vi "Get Attributes.vi"(7 "Tree ID":string, 8 "Error In":errorcluster, 10 "Attributes Names":string[](array[string]), 11 "Tree Manager":T1) -> (0 "Error Out":errorcluster, 1 "Attribute Value":variant[](array[variant]), 2 "Found?":bool[](array[boolean]), 3 "Tree Manager":T1)   [LabVIEW 2020, in "NI_VIAnCFGDataStructure.lvlib" / "Tree.lvclass"]
doc: "Get variant data attributes of the Tree."
uses:
  <vilib>/addons/analyzer/VIAnCFGDataStructure/Tree Manager/Tree.lvclass
  <vilib>/addons/analyzer/VIAnCFGDataStructure/Tree Manager/Typedefs/Session Handle.ctl
  <vilib>/addons/analyzer/VIAnCFGDataStructure/Tree Manager/Tree.lvclass/Tree.ctl
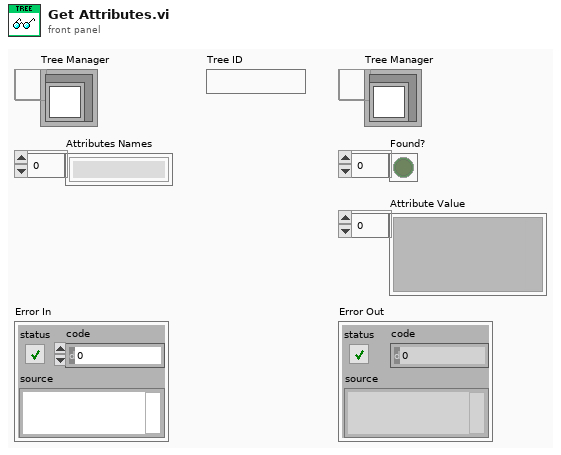
[diagram p1: front panel]
types:
  T1 = typedef "NI_VIAnCFGDataStructure.lvlib/Tree.lvclass/Session Handle.ctl" = refnum<data-value>
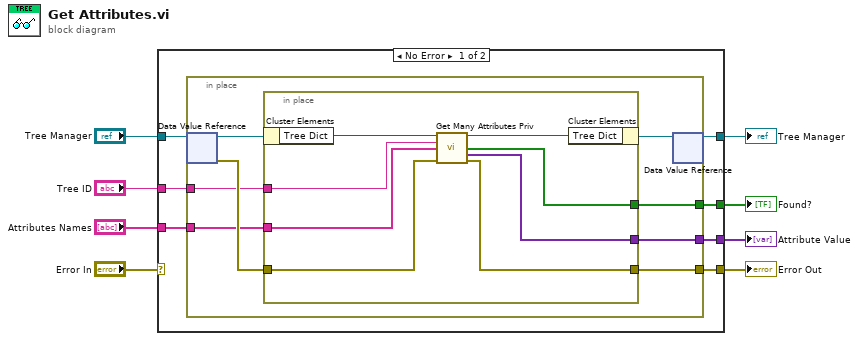
[diagram p0: block diagram]
diagram:
  n1 = case shown="No Error" "Error In" {
    selector: "Error In" -> [_ w32]
    tunnel: "Tree Manager" -> [w15 w33]
    tunnel: [w14 w33] -> w7
    tunnel: [w9 w32] -> w5
    tunnel: "Tree ID" -> [w13 _]
    tunnel: "Attributes Names" -> [w12 _]
    tunnel: [w11 _] -> w2
    tunnel: [w10 _] -> w1
    frame No Error {
      n2 = in-place {
        in-place-border: w13 -> [w20]
        in-place-border: w12 -> [w19]
        in-place-border: [w18] -> w11
        in-place-border: [w17] -> w10
        in-place-border: [w16] -> w9
        n3 = in-place-dvr #1(w15) -> (w23:refnum<class "Tree.lvclass">, w21:errorcluster)
        n4 = in-place {
          in-place-border: w21 -> [w25]
          in-place-border: w20 -> [w26]
          in-place-border: w19 -> [w27]
          in-place-border: [w29] -> w18
          in-place-border: [w28] -> w17
          in-place-border: [w24] -> w16
          n5 = in-place-cluster #2(w23) -> ("Tree Dict"=w31:variant)
          n6 = call <vilib>:"Get Many Attributes Priv.vi"("Tree Dictionary In"=w31, "Unique ID"=w26, "Attribute Names"=w27, "error in"=w25) -> ("Tree Dictionary Out"=w30:variant, "Found?"=w29:bool[], "Attribute Values"=w28:variant[], "error out"=w24:errorcluster)  [unwired: 7 in, 1 out]
          n7 = in-place-cluster #2("Tree Dict"=w30) -> (w22:refnum<class "Tree.lvclass">)
        }
        n8 = in-place-dvr #1(w22) -> (w14:T1)  [unwired: 1 out]
      }
    }
    frame Error {
    }
  }
  "Tree Manager" <- w7
  "Error Out" <- w5
  "Found?" <- w2
  "Attribute Value" <- w1
